vi "Messwerte schreiben.vi"(10 "Messdaten":sgl[](array[numeric]), 11 "Numerisch (Eingang)":i32) -> (3 "Numerisch (Ausgang)":i32)   [LabVIEW 2020, in "EPA 1065.lvlib" / "Chiller NO2 1065-376.lvlib"]
uses:
  Chiller NO2 1065-376.lvlib
  Aktion FGV Chiller Test.ctl
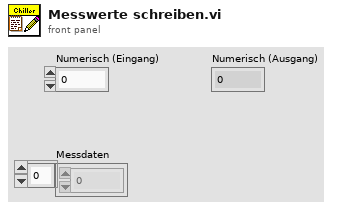
[diagram p1: front panel]
types:
  T1 = typedef "EPA 1065.lvlib/Chiller NO2 1065-376.lvlib/Aktion FGV Chiller Test.ctl" = enum16{"lesen", "Konfig Daten", "Messdaten", "Resultat", "Daten löschen", "PDF einstellen", "laden", "speichern"}
  T2 = typedef "EPA 1065.lvlib/Chiller NO2 1065-376.lvlib/Messdaten.ctl" = cluster{"xNOxRef":dbl, "xNOxmeas":dbl, "H2O":dbl, "xNOx_dry":dbl, "Bestanden":bool}
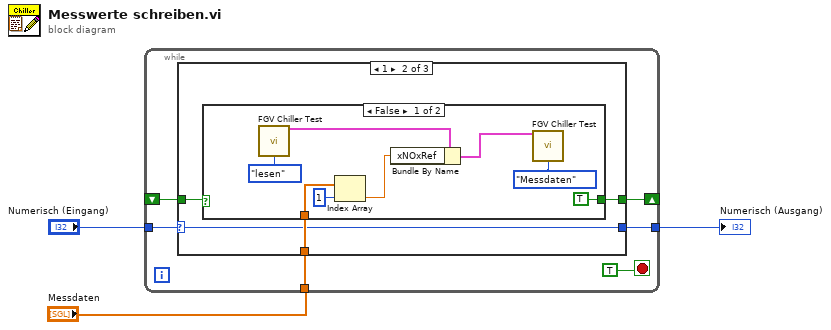
[diagram p0: block diagram]
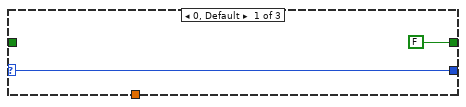
[diagram p2: hidden frame]
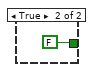
[diagram p3: hidden frame]
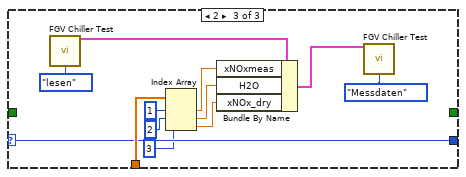
[diagram p4: hidden frame]
diagram:
  n1 = while {
    tunnel: "Messdaten" -> [w9]
    shift-right: [w7] -> _
    shift-left: _ -> [w6]
    tunnel: "Numerisch (Eingang)" -> [w5]
    tunnel: [w4] -> w1
    stop <- TRUE stop-if-true
    n2 = case shown="1" w5 {
      selector: w5 -> [w11 w14 w30]
      tunnel: w9 -> [_ w15 w32]
      tunnel: [w11 w14 w30] -> w4
      tunnel: [FALSE w12 _] -> w7
      tunnel: w6 -> [_ w13 _]
      frame 0, Default {
      }
      frame 1 {
        n3 = case shown="False" w13 {
          tunnel: w15 -> [w19 _]
          tunnel: [TRUE FALSE] -> w12
          frame False {
            n4 = call "FGV Chiller Test.vi"("Aktion"=Aktion_FGV_Chiller_Test."lesen") -> ("Daten"=w21:T2)  [unwired: 11 in, 3 out]
            n5 = Index Array(array=w19, index=1 ("Index")) -> (element=w18:sgl)
            n6 = Bundle By Name(cluster=w21, "xNOxRef"=w18) -> (w20:T2)
            n7 = call "FGV Chiller Test.vi"("Daten"=w20, "Aktion"=Aktion_FGV_Chiller_Test."Messdaten") -> ()  [unwired: 10 in, 4 out]
          }
          frame True {
          }
        }
      }
      frame 2 {
        n8 = call "FGV Chiller Test.vi"("Aktion"=Aktion_FGV_Chiller_Test."lesen") -> ("Daten"=w34:T2)  [unwired: 11 in, 3 out]
        n9 = Index Array(array=w32, index #1=1 ("Index"), index #2=2 ("Index"), index #3=3 ("Index")) -> (element #1=w31:sgl, element #2=w28:sgl, element #3=w27:sgl)
        n10 = Bundle By Name(cluster=w34, "xNOxmeas"=w31, "H2O"=w28, "xNOx_dry"=w27) -> (w33:T2)
        n11 = call "FGV Chiller Test.vi"("Daten"=w33, "Aktion"=Aktion_FGV_Chiller_Test."Messdaten") -> ()  [unwired: 10 in, 4 out]
      }
    }
  }
  "Numerisch (Ausgang)" <- w1
